vi "Target Sorting.vi"(9 "Particle Info":T2(array[cluster]), 10 "Particle scores for comparison":cluster{dbl, dbl, dbl, dbl}, 11 "Iterator":i32) -> (1 "Width":dbl, 2 "output cluster":T1, 3 "Numeric out":i32, 4 "Height":dbl, 5 "Aspect Ratio":dbl)   [LabVIEW 2012]
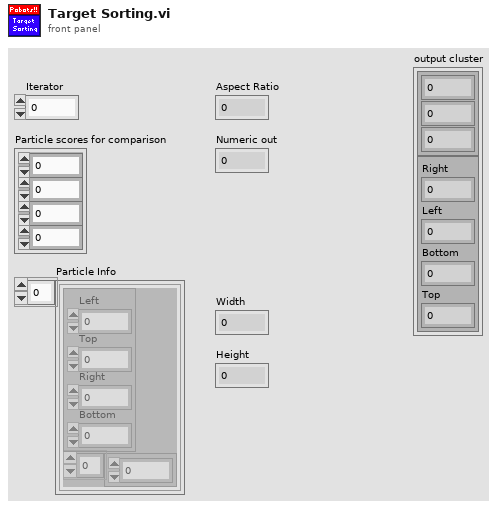
[diagram p1: front panel]
types:
  T1 = cluster{cluster{dbl, dbl, dbl}, cluster{"Right":dbl, "Left":dbl, "Bottom":dbl, "Top":dbl}}
  T2 = cluster{cluster{"Left":dbl, "Top":dbl, "Right":dbl, "Bottom":dbl}, dbl[]}[]
  T3 = cluster{"Particle Info[0]":cluster{cluster{"Left":dbl, "Top":dbl, "Right":dbl, "Bottom":dbl}, dbl[]}, "Particle Info[1]":cluster{cluster{"Left":dbl, "Top":dbl, "Right":dbl, "Bottom":dbl}, dbl[]}, "Particle Info[2]":cluster{cluster{"Left":dbl, "Top":dbl, "Right":dbl, "Bottom":dbl}, dbl[]}, "Particle Info[3]":cluster{cluster{"Left":dbl, "Top":dbl, "Right":dbl, "Bottom":dbl}, dbl[]}, "Particle Info[4]":cluster{cluster{"Left":dbl, "Top":dbl, "Right":dbl, "Bottom":dbl}, dbl[]}, "Particle Info[5]":cluster{cluster{"Left":dbl, "Top":dbl, "Right":dbl, "Bottom":dbl}, dbl[]}, "Particle Info[6]":cluster{cluster{"Left":dbl, "Top":dbl, "Right":dbl, "Bottom":dbl}, dbl[]}, "Particle Info[7]":cluster{cluster{"Left":dbl, "Top":dbl, "Right":dbl, "Bottom":dbl}, dbl[]}, "Particle Info[8]":cluster{cluster{"Left":dbl, "Top":dbl, "Right":dbl, "Bottom":dbl}, dbl[]}}
  T4 = cluster{cluster{"Left":dbl, "Top":dbl, "Right":dbl, "Bottom":dbl}, dbl[]}
  T5 = cluster{"Left":dbl, "Top":dbl, "Right":dbl, "Bottom":dbl}
  T6 = cluster{"[0]":dbl, "[1]":dbl, "[2]":dbl, "[3]":dbl, "[4]":dbl, "[5]":dbl, "[6]":dbl, "[7]":dbl, "[8]":dbl}
  T7 = cluster{"Right":dbl, "Left":dbl, "Bottom":dbl, "Top":dbl}
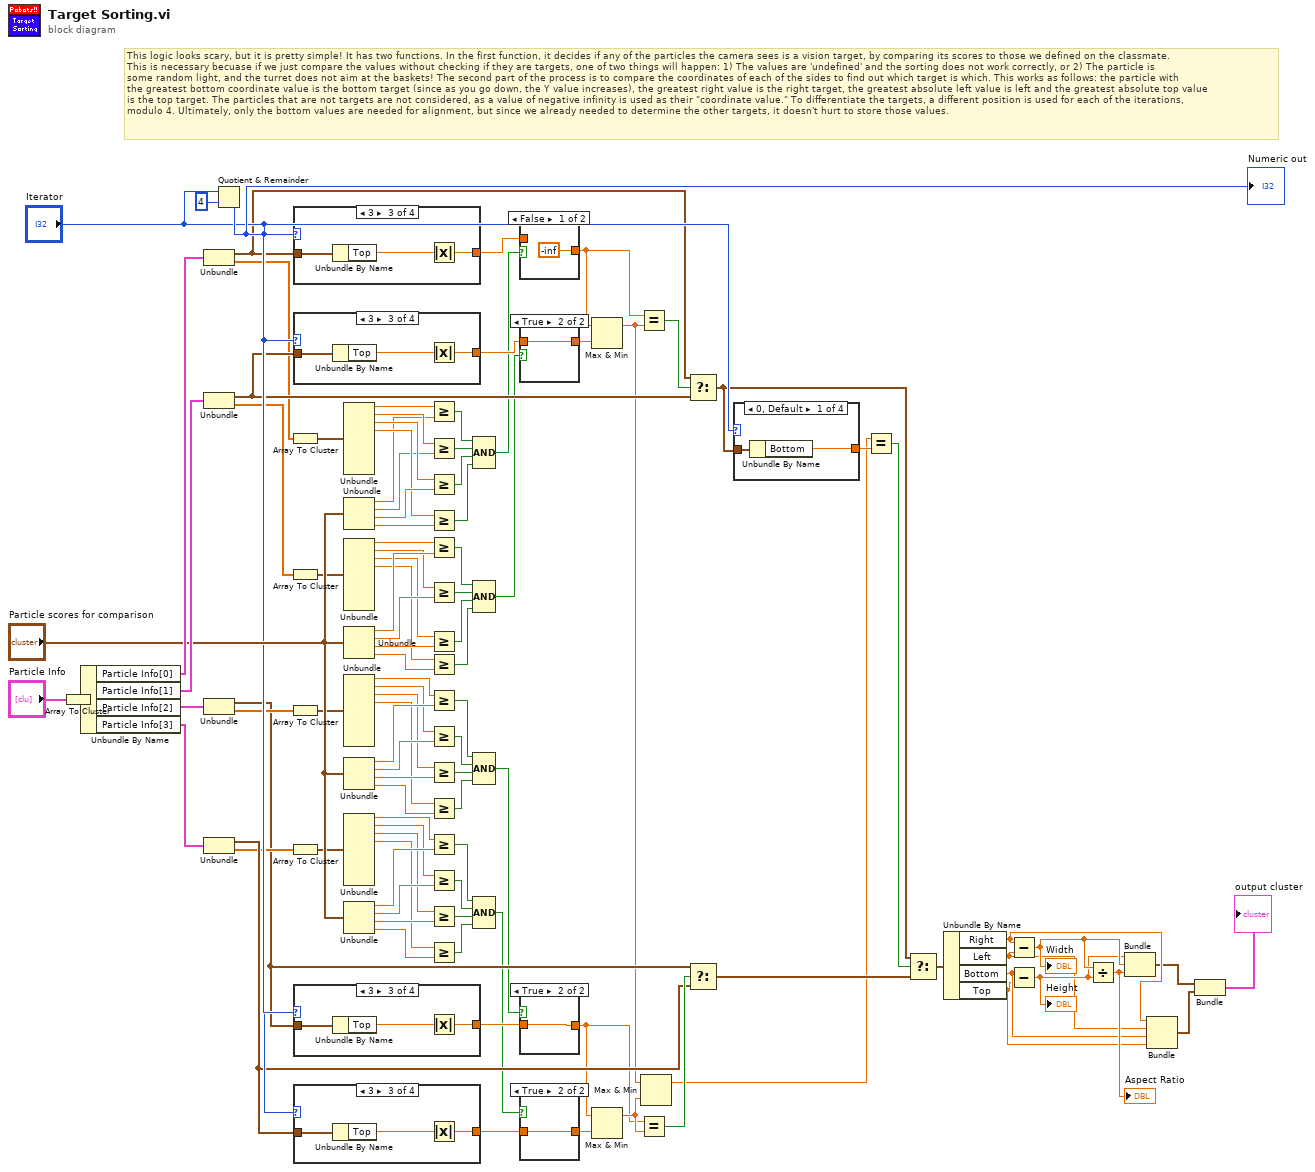
[diagram p0: block diagram]
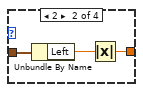
[diagram p2: hidden frame]
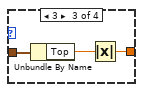
[diagram p3: hidden frame]
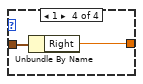
[diagram p4: hidden frame]
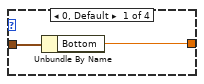
[diagram p5: hidden frame]
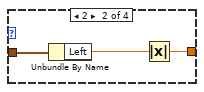
[diagram p6: hidden frame]
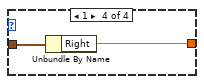
[diagram p7: hidden frame]
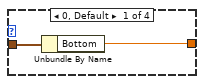
[diagram p8: hidden frame]
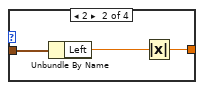
[diagram p9: hidden frame]
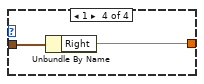
[diagram p10: hidden frame]
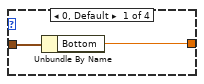
[diagram p11: hidden frame]
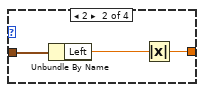
[diagram p12: hidden frame]
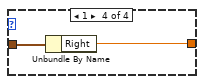
[diagram p13: hidden frame]
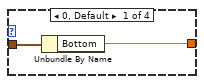
[diagram p14: hidden frame]
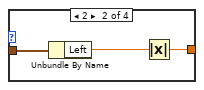
[diagram p15: hidden frame]
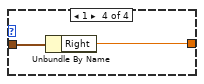
[diagram p16: hidden frame]
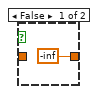
[diagram p17: hidden frame]
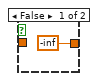
[diagram p18: hidden frame]
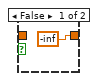
[diagram p19: hidden frame]
diagram:
  # "This logic looks scary, but it is pretty simple! It has two functions. In the first function, it decides if any of the particles the camera sees is a vision target, by comparing its scores to those we defined on the classmate.\nThis is necessary becuase if we just compare the values without checking if they are targets, one of two things will happen: 1) The values are 'undefined' and the sorting does not work correctly, or 2) The particle is \nsome random light, and the turret does not aim at the baskets! The second part of the process is to compare the coordinates of each of the sides to find out which target is which. This works as follows: the particle with\nthe greatest bottom coordinate value is the bottom target (since as you go down, the Y value increases), the greatest right value is the right target, the greatest absolute left value is left and the greatest absolute top value\nis the top target. The particles that are not targets are not considered, as a value of negative infinity is used as their \"coordinate value.\" To differentiate the targets, a different position is used for each of the iterations,\nmodulo 4. Ultimately, only the bottom values are needed for alignment, but since we already needed to determine the other targets, it doesn't hurt to store those values."
  n1 = Array To Cluster(array="Particle Info") -> (cluster=w79:T3)
  n2 = Unbundle By Name(w79) -> ("Particle Info[0]"=w96:T4, "Particle Info[1]"=w97:T4, "Particle Info[2]"=w98:T4, "Particle Info[3]"=w99:T4)
  n3 = Unbundle(w96) -> (w85:T5, w22:dbl[])
  n4 = Unbundle(w97) -> (w83:T5, w23:dbl[])
  n5 = Unbundle(w98) -> (w18:T5, w24:dbl[])
  n6 = Unbundle(w99) -> (w81:T5, w25:dbl[])
  n7 = Quotient & Remainder(x="Iterator", y=4) -> (x-y*floor(x/y)=w93:i32)  [unwired: 1 out]
  "Numeric out" <- w93
  n8 = Array To Cluster(array=w22) -> (cluster=w26:T6)
  n9 = Array To Cluster(array=w23) -> (cluster=w27:T6)
  n10 = Array To Cluster(array=w24) -> (cluster=w28:T6)
  n11 = Array To Cluster(array=w25) -> (cluster=w29:T6)
  n12 = case shown="3" "Iterator" {
    tunnel: [w103 w105 w108 w112] -> w86
    tunnel: w85 -> [w104 w106 w109 w111]
    frame 0, Default {
      n13 = Unbundle By Name(w104) -> ("Bottom"=w103:dbl)
    }
    frame 2 {
      n14 = Unbundle By Name(w106) -> ("Left"=w107:dbl)
      n15 = Absolute Value(x=w107) -> (abs(x)=w105:dbl)
    }
    frame 3 {
      n16 = Unbundle By Name(w109) -> ("Top"=w110:dbl)
      n17 = Absolute Value(x=w110) -> (abs(x)=w108:dbl)
    }
    frame 1 {
      n18 = Unbundle By Name(w111) -> ("Right"=w112:dbl)
    }
  }
  n19 = case shown="3" "Iterator" {
    tunnel: [w113 w115 w118 w122] -> w84
    tunnel: w83 -> [w114 w116 w119 w121]
    frame 0, Default {
      n20 = Unbundle By Name(w114) -> ("Bottom"=w113:dbl)
    }
    frame 2 {
      n21 = Unbundle By Name(w116) -> ("Left"=w117:dbl)
      n22 = Absolute Value(x=w117) -> (abs(x)=w115:dbl)
    }
    frame 3 {
      n23 = Unbundle By Name(w119) -> ("Top"=w120:dbl)
      n24 = Absolute Value(x=w120) -> (abs(x)=w118:dbl)
    }
    frame 1 {
      n25 = Unbundle By Name(w121) -> ("Right"=w122:dbl)
    }
  }
  n26 = case shown="3" w93 {
    tunnel: [w123 w125 w128 w132] -> w14
    tunnel: w18 -> [w124 w126 w129 w131]
    frame 0, Default {
      n27 = Unbundle By Name(w124) -> ("Bottom"=w123:dbl)
    }
    frame 2 {
      n28 = Unbundle By Name(w126) -> ("Left"=w127:dbl)
      n29 = Absolute Value(x=w127) -> (abs(x)=w125:dbl)
    }
    frame 3 {
      n30 = Unbundle By Name(w129) -> ("Top"=w130:dbl)
      n31 = Absolute Value(x=w130) -> (abs(x)=w128:dbl)
    }
    frame 1 {
      n32 = Unbundle By Name(w131) -> ("Right"=w132:dbl)
    }
  }
  n33 = case shown="3" "Iterator" {
    tunnel: [w133 w135 w138 w142] -> w82
    tunnel: w81 -> [w134 w136 w139 w141]
    frame 0, Default {
      n34 = Unbundle By Name(w134) -> ("Bottom"=w133:dbl)
    }
    frame 2 {
      n35 = Unbundle By Name(w136) -> ("Left"=w137:dbl)
      n36 = Absolute Value(x=w137) -> (abs(x)=w135:dbl)
    }
    frame 3 {
      n37 = Unbundle By Name(w139) -> ("Top"=w140:dbl)
      n38 = Absolute Value(x=w140) -> (abs(x)=w138:dbl)
    }
    frame 1 {
      n39 = Unbundle By Name(w141) -> ("Right"=w142:dbl)
    }
  }
  n40 = Unbundle(w26) -> ("[0]"=w30:dbl, "[1]"=w33:dbl, "[2]"=w34:dbl, "[3]"=w35:dbl)  [unwired: 5 out]
  n41 = Unbundle("Particle scores for comparison") -> (w31:dbl, w32:dbl, w36:dbl, w37:dbl)
  n42 = Unbundle(w27) -> ("[0]"=w38:dbl, "[1]"=w39:dbl, "[2]"=w40:dbl, "[3]"=w41:dbl)  [unwired: 5 out]
  n43 = Unbundle("Particle scores for comparison") -> (w42:dbl, w43:dbl, w44:dbl, w45:dbl)
  n44 = Unbundle(w28) -> ("[0]"=w46:dbl, "[1]"=w47:dbl, "[2]"=w48:dbl, "[3]"=w49:dbl)  [unwired: 5 out]
  n45 = Unbundle("Particle scores for comparison") -> (w50:dbl, w51:dbl, w52:dbl, w53:dbl)
  n46 = Unbundle(w29) -> ("[0]"=w54:dbl, "[1]"=w55:dbl, "[2]"=w56:dbl, "[3]"=w57:dbl)  [unwired: 5 out]
  n47 = Unbundle("Particle scores for comparison") -> (w58:dbl, w59:dbl, w60:dbl, w61:dbl)
  n48 = Greater Or Equal?(x=w30, y=w31) -> (x >= y?=w62:bool)
  n49 = Greater Or Equal?(x=w33, y=w32) -> (x >= y?=w63:bool)
  n50 = Greater Or Equal?(x=w34, y=w36) -> (x >= y?=w64:bool)
  n51 = Greater Or Equal?(x=w35, y=w37) -> (x >= y?=w65:bool)
  n52 = Greater Or Equal?(x=w38, y=w42) -> (x >= y?=w77:bool)
  n53 = Greater Or Equal?(x=w39, y=w43) -> (x >= y?=w76:bool)
  n54 = Greater Or Equal?(x=w40, y=w44) -> (x >= y?=w75:bool)
  n55 = Greater Or Equal?(x=w41, y=w45) -> (x >= y?=w74:bool)
  n56 = Greater Or Equal?(x=w46, y=w50) -> (x >= y?=w73:bool)
  n57 = Greater Or Equal?(x=w47, y=w51) -> (x >= y?=w72:bool)
  n58 = Greater Or Equal?(x=w48, y=w52) -> (x >= y?=w71:bool)
  n59 = Greater Or Equal?(x=w49, y=w53) -> (x >= y?=w70:bool)
  n60 = Greater Or Equal?(x=w54, y=w58) -> (x >= y?=w66:bool)
  n61 = Greater Or Equal?(x=w55, y=w59) -> (x >= y?=w67:bool)
  n62 = Greater Or Equal?(x=w56, y=w60) -> (x >= y?=w68:bool)
  n63 = Greater Or Equal?(x=w57, y=w61) -> (x >= y?=w69:bool)
  n64 = Compound Arithmetic op=AND(w62, w63, w64, w65) -> (w8:bool)
  n65 = Compound Arithmetic op=AND(w77, w76, w75, w74) -> (w9:bool)
  n66 = Compound Arithmetic op=AND(w73, w72, w71, w70) -> (w10:bool)
  n67 = Compound Arithmetic op=AND(w66, w67, w68, w69) -> (w11:bool)
  n68 = case shown="False" w8 {
    tunnel: [-inf w144] -> w15
    tunnel: w86 -> [_ w144]
    frame False {
    }
    frame True {
    }
  }
  n69 = case shown="True" w9 {
    tunnel: [-inf w146] -> w12
    tunnel: w84 -> [_ w146]
    frame False {
    }
    frame True {
    }
  }
  n70 = case shown="True" w10 {
    tunnel: [-inf w148] -> w17
    tunnel: w14 -> [_ w148]
    frame False {
    }
    frame True {
    }
  }
  n71 = case shown="True" w11 {
    tunnel: [-inf w150] -> w13
    tunnel: w82 -> [_ w150]
    frame False {
    }
    frame True {
    }
  }
  n72 = Max & Min(x=w15, y=w12) -> (max(x,y)=w16:dbl)  [unwired: 1 out]
  n73 = Max & Min(x=w17, y=w13) -> (max(x,y)=w102:dbl)  [unwired: 1 out]
  n74 = Equal?(x=w15, y=w16) -> (x = y?=w95:bool)
  n75 = Equal?(x=w17, y=w102) -> (x = y?=w100:bool)
  n76 = Max & Min(x=w16, y=w102) -> (max(x,y)=w19:dbl)  [unwired: 1 out]
  n77 = Select(t=w85, s=w95, f=w83) -> (s? t:f=w87:T5)
  n78 = Select(t=w18, s=w100, f=w81) -> (s? t:f=w20:T5)
  n79 = case shown="0, Default" "Iterator" {
    tunnel: [w151 w153 w156 w160] -> w88
    tunnel: w87 -> [w152 w154 w157 w159]
    frame 0, Default {
      n80 = Unbundle By Name(w152) -> ("Bottom"=w151:dbl)
    }
    frame 2 {
      n81 = Unbundle By Name(w154) -> ("Left"=w155:dbl)
      n82 = Absolute Value(x=w155) -> (abs(x)=w153:dbl)
    }
    frame 3 {
      n83 = Unbundle By Name(w157) -> ("Top"=w158:dbl)
      n84 = Absolute Value(x=w158) -> (abs(x)=w156:dbl)
    }
    frame 1 {
      n85 = Unbundle By Name(w159) -> ("Right"=w160:dbl)
    }
  }
  n86 = Equal?(x=w19, y=w88) -> (x = y?=w101:bool)
  n87 = Select(t=w87, s=w101, f=w20) -> (s? t:f=w21:T5)
  n88 = Unbundle By Name(w21) -> ("Right"=w7:dbl, "Left"=w6:dbl, "Bottom"=w5:dbl, "Top"=w4:dbl)
  n89 = Subtract(x=w7, y=w6) -> (x-y=w91:dbl)
  "Width" <- w91
  n90 = Subtract(x=w5, y=w4) -> (x-y=w90:dbl)
  "Height" <- w90
  n91 = Divide(x=w91, y=w90) -> (x/y=w92:dbl)
  "Aspect Ratio" <- w92
  n92 = Bundle(w90, w91, w92) -> (w3:cluster{dbl, dbl, dbl})  [unwired: 1 in]
  n93 = Bundle("Right"=w7, "Left"=w6, "Bottom"=w5, "Top"=w4) -> (w2:T7)  [unwired: 1 in]
  n94 = Bundle(w3, w2) -> (→"output cluster":T1)  [unwired: 1 in]
